vi "DefBallEnemySkill.vi"(8 "error in (no error)":errorcluster, 9 "Robot":refnum<class "Robot.lvclass">, 10 "Game":refnum<class "Game.lvclass">, 11 "DefBallEnemySkill in":refnum<class "DefBallEnemySkill.lvclass">) -> (0 "error out":errorcluster, 2 "robot out":refnum<class "Robot.lvclass">, 3 "DefBallEnemySkill out":refnum<class "DefBallEnemySkill.lvclass">)   [LabVIEW 2023, in "DefBallEnemySkill.lvclass"]
uses:
  DefBallEnemySkill.lvclass
  Robot_class/Robot.lvclass
  Game_class/Game.lvclass
  Utilities_class/Utilities.lvclass
  Game_class/Game.lvclass/Game.ctl
  Referee_class/Referee.lvclass/Referee.ctl
  Parameters_class/Parameters.lvclass/Parameters.ctl
  Team_class/Team.lvclass/Team.ctl
  Object_class/Object.lvclass/Object.ctl
  Robot_class/Robot.lvclass/Robot.ctl
  Game_class/Read Parameters.lvclass.vi
  Game_class/Read BallRef.vi
  Parameters_class/Read AttakingOurselves.vi
  Game_class/Read AllyRef.vi
  Game_class/Read EnemyRef.vi
  Object_class/Read x.vi
  Object_class/Read y.vi
  Team_class/Read RobotRef.vi
  Game_class/Read Referee.vi
  Game_class/Read FieldRef.vi
  Game_class/Read Utilities.lvclass.vi
  Parameters_class/Read GoalieInFrontGoal.vi
  Referee_class/Read our_goalie_id.vi
  Robot_class/Write dest_x.vi
  Robot_class/Write dest_y.vi
  Robot_class/Write dest_orientation.vi
  Ball_class/Ball.lvclass
  Enemy_class/Enemy.lvclass
  Ally_class/Ally.lvclass
  Referee_class/Referee.lvclass
  Field_class/Field.lvclass
  Parameters_class/Parameters.lvclass
panel:
  in  "goalie distance from goal line":dbl=150.0
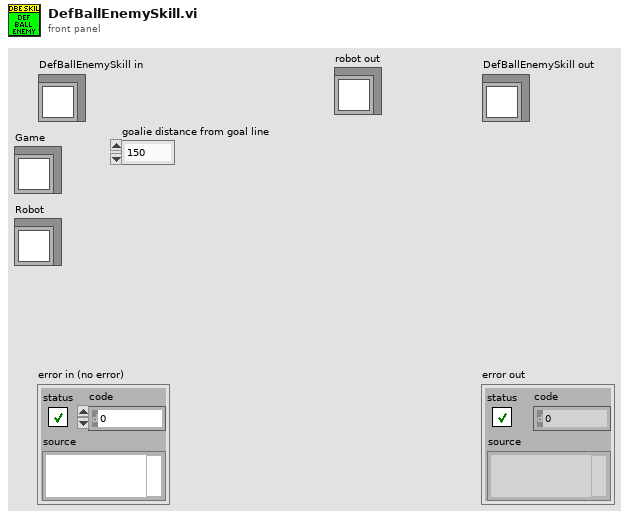
[diagram p1: front panel]
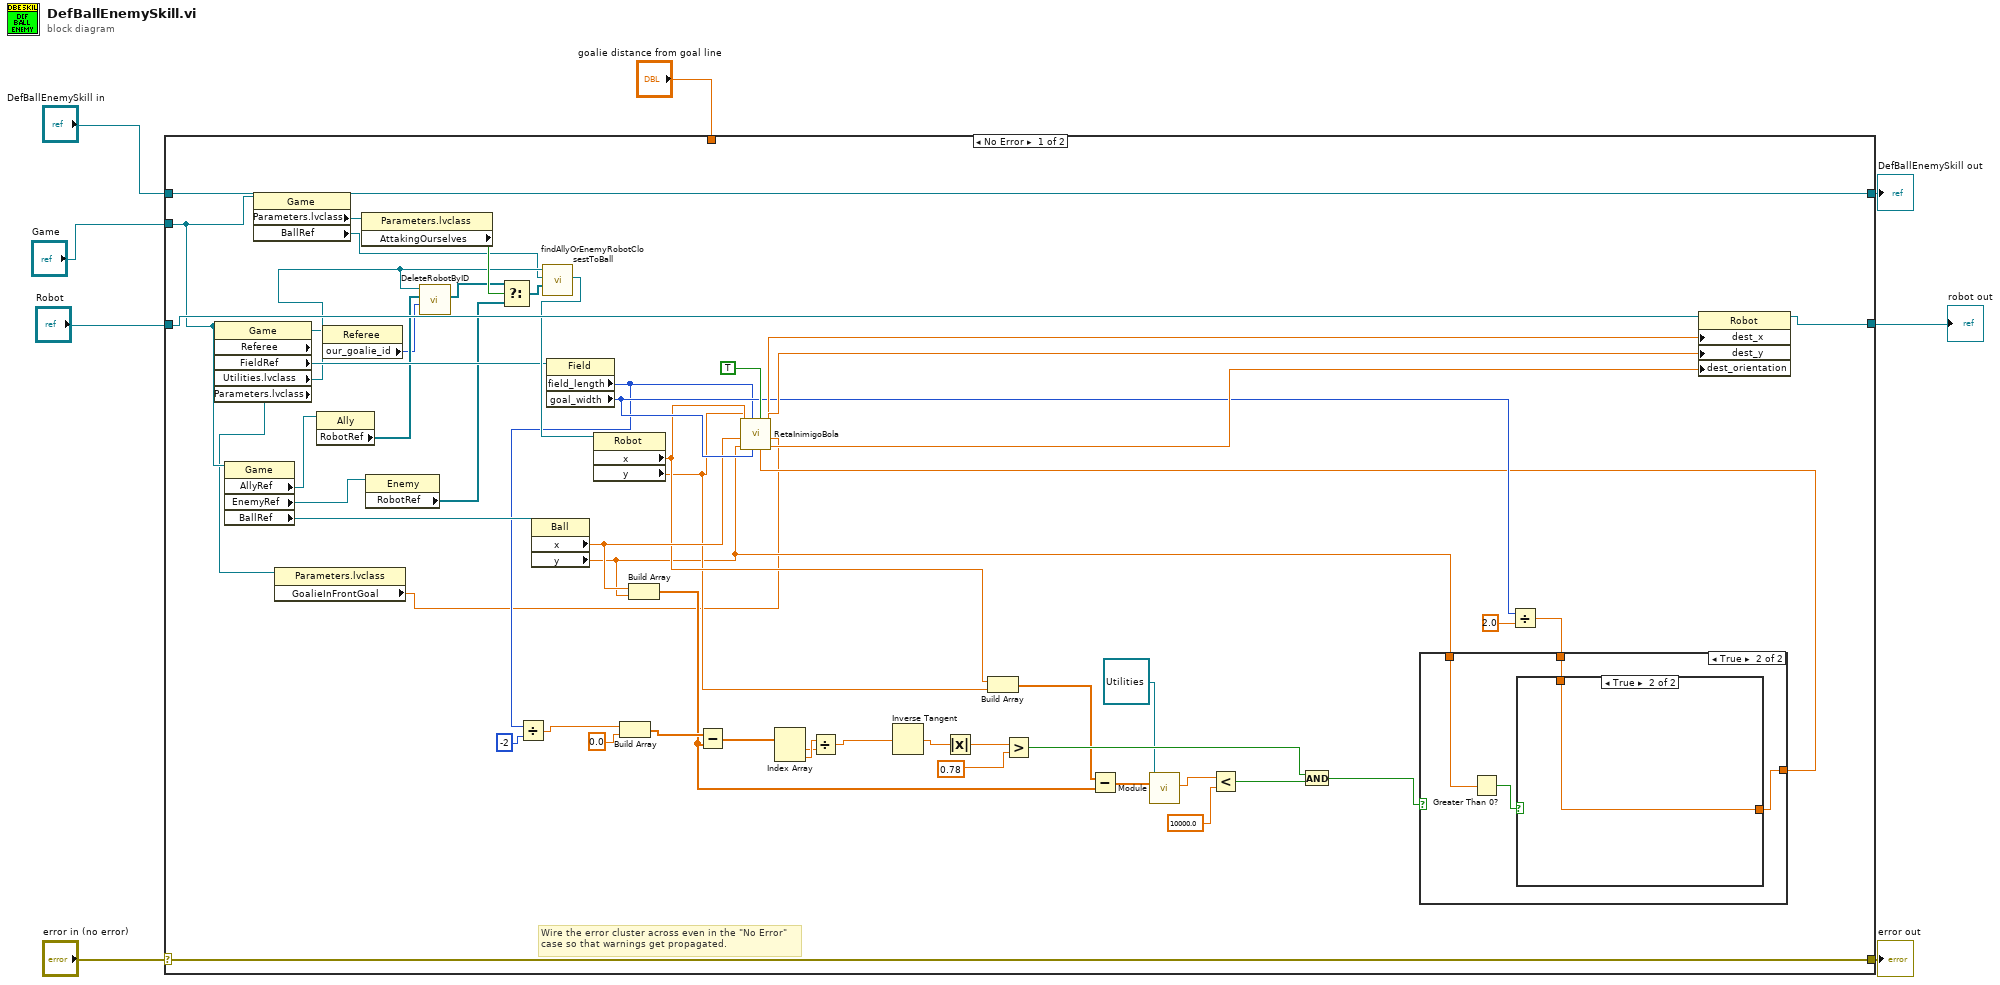
[diagram p0: block diagram]
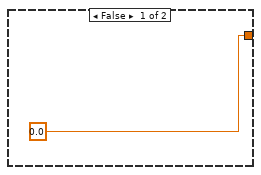
[diagram p2: hidden frame]
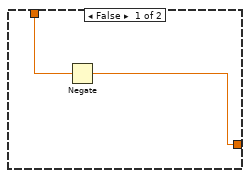
[diagram p3: hidden frame]
diagram:
  n1 = case shown="No Error" "error in (no error)" {
    selector: "error in (no error)" -> [w62 w73]
    tunnel: [w62 w73] -> w7
    tunnel: [w63 w72] -> w5
    tunnel: "DefBallEnemySkill in" -> [w63 w72]
    tunnel: "Robot" -> [w61 _]
    tunnel: "Game" -> [w23 _]
    tunnel: "goalie distance from goal line" -> [_ _]
    tunnel: [w25 _] -> w1
    frame No Error {
      # "Wire the error cluster across even in the \"No Error\"\ncase so that warnings get propagated."
      n2 = property class="Game"(reference=w23) -> ("Referee"=w15:refnum<class "Referee.lvclass">, "FieldRef"=w58:refnum<class "Field.lvclass">, "Utilities.lvclass"=w17:refnum<class "Utilities.lvclass">, "Parameters.lvclass"=w11:refnum<class "Parameters.lvclass">)  [unwired: 1 in, 2 out]
      n3 = property class="Game"(reference=w23) -> ("AllyRef"=w18:refnum<class "Ally.lvclass">, "EnemyRef"=w20:refnum<class "Enemy.lvclass">, "BallRef"=w59:refnum<class "Ball.lvclass">)  [unwired: 1 in, 2 out]
      n4 = property class="Game"(reference=w23) -> ("Parameters.lvclass"=w22:refnum<class "Parameters.lvclass">, "BallRef"=w9:refnum<class "Ball.lvclass">)  [unwired: 1 in, 2 out]
      n5 = property class="Parameters.lvclass"(reference=w11) -> ("GoalieInFrontGoal"=w10:dbl)  [unwired: 1 in, 2 out]
      n6 = property class="Ally"(reference=w18) -> ("RobotRef"=w16:refnum<class "Robot.lvclass">[])  [unwired: 1 in, 2 out]
      n7 = property class="Referee"(reference=w15) -> ("our_goalie_id"=w14:i32)  [unwired: 1 in, 2 out]
      n8 = property class="Parameters.lvclass"(reference=w22) -> ("AttakingOurselves"=w21:bool)  [unwired: 1 in, 2 out]
      n9 = property class="Enemy"(reference=w20) -> ("RobotRef"=w19:refnum<class "Robot.lvclass">[])  [unwired: 1 in, 2 out]
      n10 = call-dynamic "DeleteRobotByID.vi"("id"=w14, "RobotRef"=w16, "Utilities in"=w17) -> ("RobotRef out"=w13:refnum<class "Robot.lvclass">[])  [unwired: 6 in, 2 out]
      n11 = Select(t=w13, s=w21, f=w19) -> (s? t:f=w12:refnum<class "Robot.lvclass">[])
      n12 = property class="Ball"(reference=w59) -> ("x"=w38:dbl, "y"=w26:dbl)  [unwired: 1 in, 2 out]
      n13 = call "findAllyOrEnemyRobotClosestToBall.vi"("Ally/Enemy Robots"=w12, "Ball"=w9, "Utilities in"=w17) -> ("Robot"=w60:refnum<class "Robot.lvclass">)  [unwired: 5 in, 3 out]
      n14 = property class="Field"(reference=w58) -> ("field_length"=w39:i32, "goal_width"=w51:i32)  [unwired: 1 in, 2 out]
      n15 = Divide(x=w39, y=-2) -> (x/y=w45:dbl)
      n16 = property class="Robot"(reference=w60) -> ("x"=w31:dbl, "y"=w30:dbl)  [unwired: 1 in, 2 out]
      n17 = Build Array(w45, 0.0 ("element")) -> (w48:dbl[])
      n18 = Build Array(w38, w26) -> (w28:dbl[])
      n19 = Subtract(x=w48, y=w28) -> (x-y=w47:dbl[])
      n20 = Index Array(array=w47) -> (element #1=w43:dbl, element #2=w44:dbl)  [unwired: 2 in]
      n21 = Divide(x=w44, y=w43) -> (x/y=w42:dbl)
      n22 = Inverse Tangent(1:w42) -> (0:w41:dbl)
      n23 = Absolute Value(x=w41) -> (abs(x)=w46:dbl)
      n24 = Build Array(w31, w30) -> (w29:dbl[])
      n25 = Greater?(x=w46, y=0.78) -> (0:w35:bool)
      n26 = Subtract(x=w29, y=w28) -> (x-y=w33:dbl[])
      n27 = call-dynamic "Module.vi"("2D vector"=w33, "Utilities in"=refnum<class "Utilities.lvclass"> refnum) -> ("Modulo"=w32:dbl)  [unwired: 7 in, 2 out]
      n28 = Less?(x=w32, y=10000.0) -> (x < y?=w36:bool)
      n29 = And(x=w35, y=w36) -> (x .and. y?=w34:bool)
      n30 = Divide(x=w51, y=2.0) -> (x/y=w53:dbl)
      n31 = case shown="True" w34 {
        tunnel: w53 -> [_ w67]
        tunnel: [0.0 w66] -> w27
        tunnel: w26 -> [_ w65]
        frame False {
        }
        frame True {
          n32 = Greater Than 0?(x=w65) -> (x > 0?=w68:bool)
          n33 = case shown="True" w68 {
            tunnel: w67 -> [w70 w71]
            tunnel: [w69 w71] -> w66
            frame False {
              n34 = Negate(x=w70) -> (-x=w69:dbl)
            }
            frame True {
            }
          }
        }
      }
      n35 = call "RetaInimigoBola.vi"("DistInFrontGoal"=w10, "Y quina"=w27, "Meio?"=TRUE, "Goal width"=w51, "Field lenght"=w39, "Y bola"=w26, "X bola"=w38, "Y inimigo"=w30, "X inimigo"=w31) -> ("Orientação"=w55:dbl, "Y goleiro"=w57:dbl, "X goleiro"=w56:dbl)
      n36 = property class="Robot"(reference=w61, "dest_x"=w56, "dest_y"=w57, "dest_orientation"=w55) -> (reference out=w25:refnum<class "Robot.lvclass">)  [unwired: 1 in, 1 out]
    }
    frame Error {
    }
  }
  "error out" <- w7
  "DefBallEnemySkill out" <- w5
  "robot out" <- w1
